vi "clear arduino parse error (sub-vi).vi"(8 "error in":errorcluster) -> (0 "error out":errorcluster)   [LabVIEW 2021]
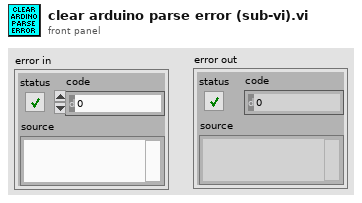
[diagram p1: front panel]
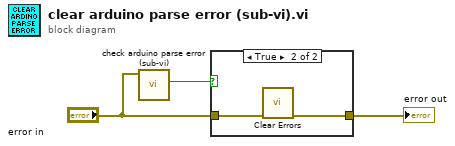
[diagram p0: block diagram]
diagram:
  n1 = call "check arduino parse error (sub-vi).vi"("error"="error in") -> ("is arduino parse error?"=w3:bool)  [unwired: 10 in]
  n2 = case shown="True" w3 {
    tunnel: "error in" -> [w4 w6]
    tunnel: [w4 w5] -> w1
    frame False {
    }
    frame True {
      n3 = call <vilib>:"Clear Errors.vi"("error in (no error)"=w6) -> ("error out"=w5:errorcluster)  [unwired: 5 in, 1 out]
    }
  }
  "error out" <- w1
